vi "GET_2D_Data_Binning_(additional_data).vi"(3 "Additional data":dbl[](array[numeric]), 4 "Y":dbl[](array[numeric]), 5 "X":dbl[](array[numeric]), 6 "Bins parameters":T1={"Xmax"=110.0, "Xmin"=-110.0, "Ymax"=110.0, "Ymin"=-110.0, "# bins per axis"=64}) -> (2 "Binned array":dbl[][](array[numeric]))   [LabVIEW 2018, in "Tracker.lvlib"]
uses:
  Tracker.lvlib
  Controls/CTL_2D_bins_parameters.ctl
  Common_Resources.lvlib
panel:
  out "Counts array":u32[][](array[numeric])
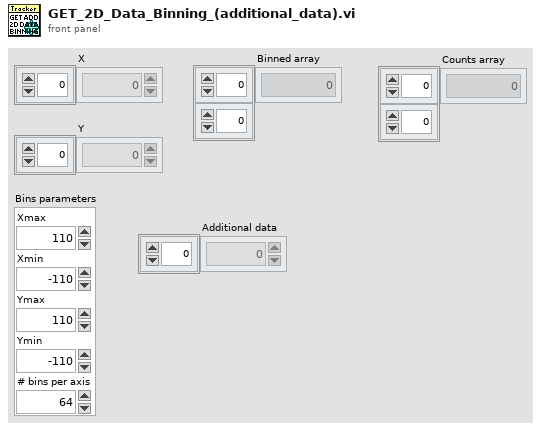
[diagram p1: front panel]
types:
  T1 = typedef "Common_Resources.lvlib/CTL_2D_bins_parameters.ctl" = cluster{"Xmax":dbl, "Xmin":dbl, "Ymax":dbl, "Ymin":dbl, "# bins per axis":i32}
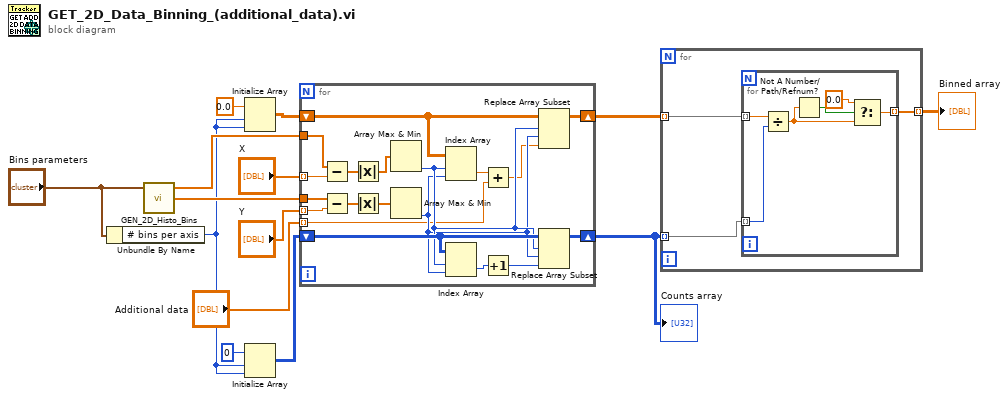
[diagram p0: block diagram]
diagram:
  n1 = Unbundle By Name("Bins parameters") -> ("# bins per axis"=w6:i32)
  n2 = call "GEN_2D_Histo_Bins.vi"("Bins parameters"="Bins parameters") -> ("Y bins (center)"=w13:dbl[], "X bins (center)"=w14:dbl[])  [unwired: 2 in, 1 out]
  n3 = Initialize Array(0.0, w6, w6) -> (w5:dbl[][])
  n4 = Initialize Array(u32 0, w6, w6) -> (w11:u32[][])
  n5 = for {
    tunnel: "X" -> [w32] mode=indexing
    tunnel: "Y" -> [w29] mode=indexing
    tunnel: w14 -> [w33]
    tunnel: w13 -> [w28]
    shift-right: [w25] -> w2
    shift-left: w11 -> [w27]
    shift-right: [w18] -> w3
    shift-left: w5 -> [w19]
    tunnel: "Additional data" -> [w16] mode=indexing
    n6 = Subtract(x=w33, y=w32) -> (x-y=w31:dbl[])
    n7 = Subtract(x=w28, y=w29) -> (x-y=w30:dbl[])
    n8 = Absolute Value(x=w31) -> (abs(x)=w23:dbl[])
    n9 = Absolute Value(x=w30) -> (abs(x)=w22:dbl[])
    n10 = Array Max & Min(array=w23) -> (min index (indices)=w21:i32)  [unwired: 3 out]
    n11 = Array Max & Min(array=w22) -> (min index (indices)=w20:i32)  [unwired: 3 out]
    n12 = Index Array(array=w19, index (row)=w21, index (col)=w20) -> (element=w17:dbl)
    n13 = Index Array(array=w27, index (row)=w21, index (col)=w20) -> (element=w26:u32)
    n14 = Add(x=w17, y=w16) -> (x+y=w15:dbl)
    n15 = Increment(x=w26) -> (x+1=w24:u32)
    n16 = Replace Array Subset(array=w19, new element=w15, index (row)=w21, index (col)=w20) -> (w18:dbl[][])
    n17 = Replace Array Subset(array=w27, new element=w24, index (row)=w21, index (col)=w20) -> (w25:u32[][])
  }
  "Counts array" <- w2
  n18 = for {
    tunnel: w3 -> [w36] mode=indexing
    tunnel: w2 -> [w35] mode=indexing
    tunnel: [w34] -> w1 mode=indexing
    n19 = for {
      tunnel: w36 -> [w42] mode=indexing
      tunnel: w35 -> [w41] mode=indexing
      tunnel: [w37] -> w34 mode=indexing
      n20 = Divide(x=w42, y=w41) -> (x/y=w39:dbl)
      n21 = Not A Number/Path/Refnum?(number/path/refnum=w39) -> (NaN/Path/Refnum?=w40:bool)
      n22 = Select(t=0.0, s=w40, f=w39) -> (s? t:f=w37:dbl)
    }
  }
  "Binned array" <- w1
